vi "Sort Fcurve.vi"(0 "reference in":refnum<class "Force Curve_tdms.lvclass">, 5 "error in (no error)":errorcluster) -> (14 "reference out":refnum<class "Force Curve_tdms.lvclass">, 19 "error out":errorcluster)   [LabVIEW 2019, in "Force Curve_tdms.lvclass"]
uses:
  Force Curve_tdms.lvclass
  Signal In.ctl
  TDMS_DataHandler_class/property name combo box.ctl
  TDMS_DataHandler_class/TDMS_DataHandler.lvclass
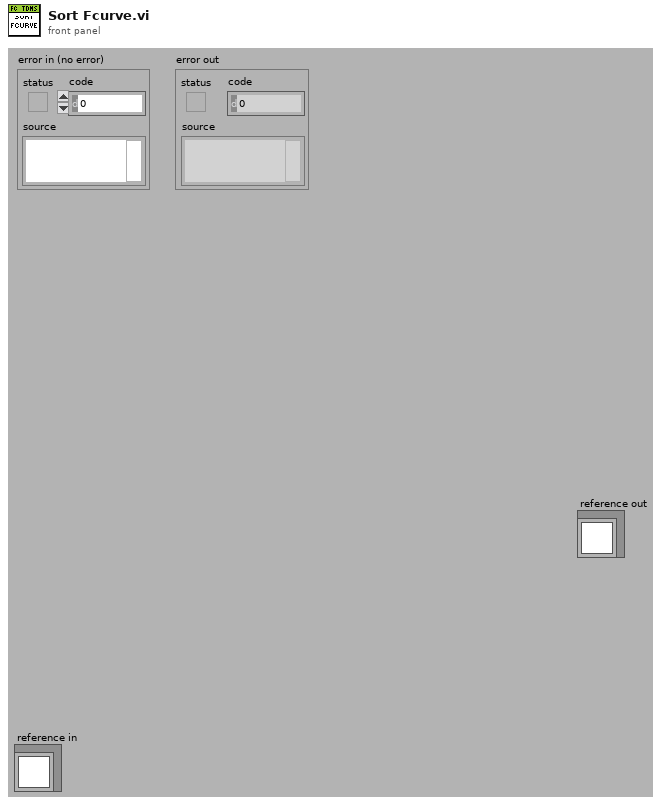
[diagram p1: front panel]
types:
  T1 = typedef "Force Curve_tdms.lvclass/Signal In.ctl" = enum16{"Deflection", "SensorIn", "MockOut", "ZstageOut"}
  T2 = typedef "TDMS_DataHandler.lvclass/property name combo box.ctl" = string
  T3 = typedef "Force Curve_tdms.lvclass/Fcurve Meta data analysis.ctl" = cluster{"dt (us)":dbl, "Dec Factor":dbl, "Z piezo Sensitivity (nm/V)":dbl, "K (N/m)":dbl, "Sp (V)":dbl, "Contact (ms)":dbl, "Zpos contact":dbl, "Vel_app (nm/s)":dbl, "Vel_ret (nm/s)":dbl, "deltaV (nm)":dbl, "Def_V0 (v)":dbl, "Decimating Factor":dbl}
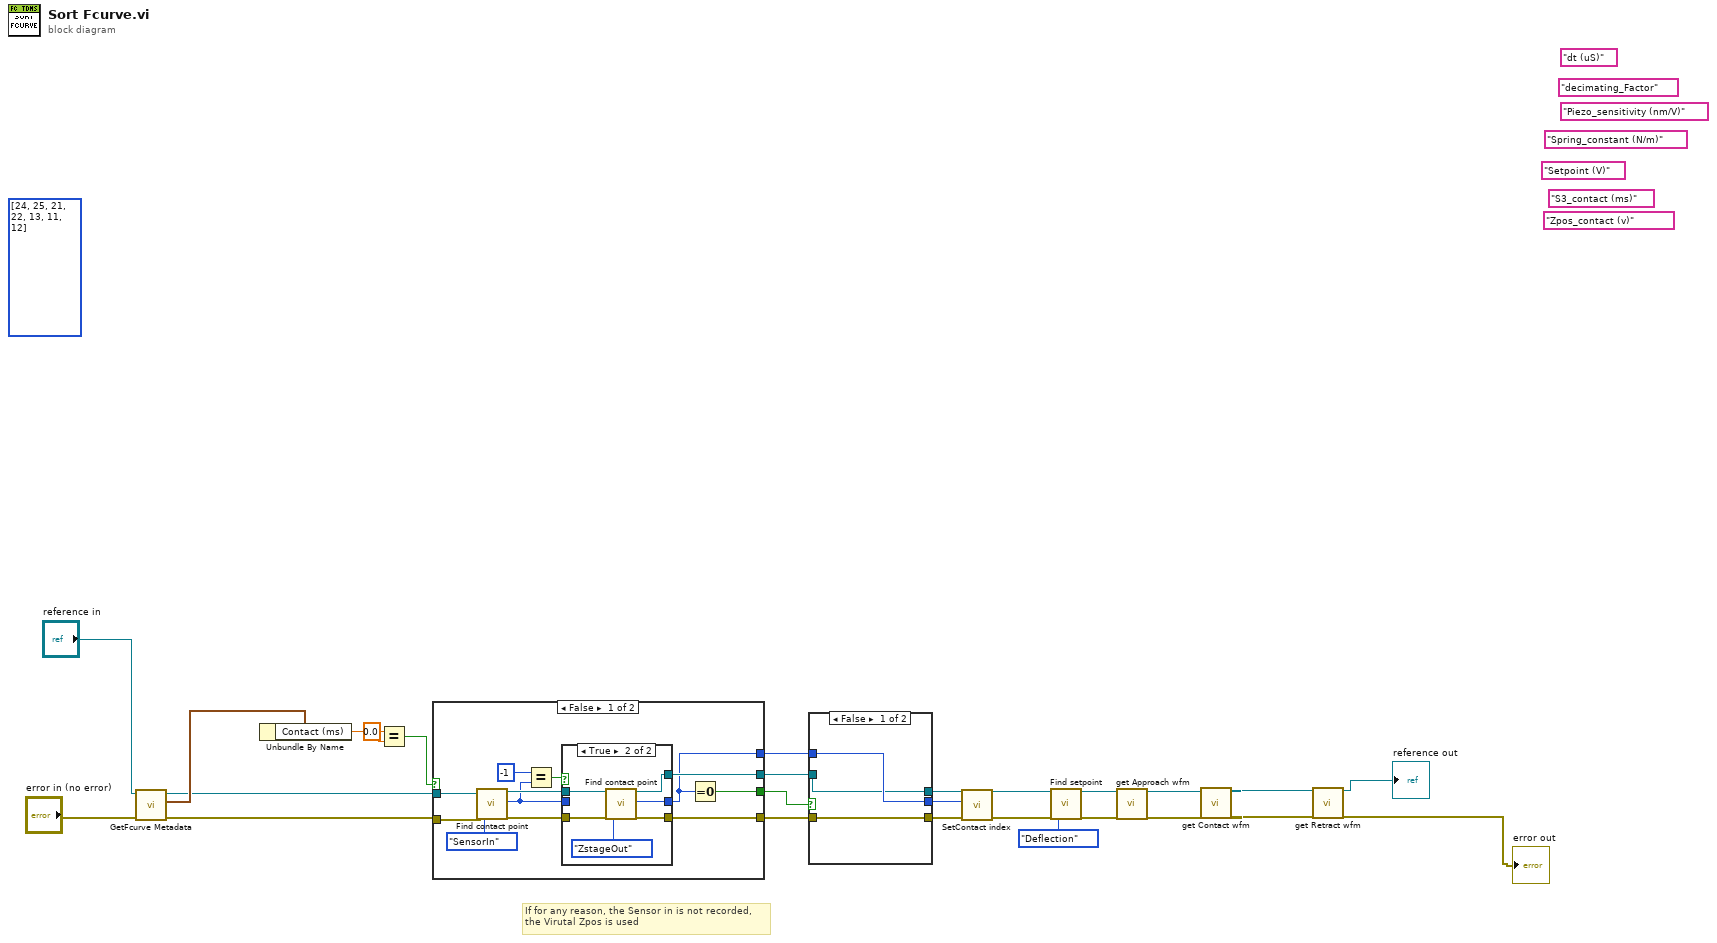
[diagram p0: block diagram]
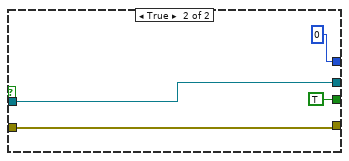
[diagram p3: hidden frame]
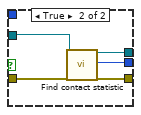
[diagram p4: hidden frame]
diagram:
  (unwired) i32[] [24, 25, 21, 22, 13, 11, 12] ("Array")
  (unwired) T2 "Setpoint (V)" ("Combo Box")
  (unwired) T2 "S3_contact (ms)" ("Combo Box")
  (unwired) T2 "Zpos_contact (v)" ("Combo Box")
  (unwired) T2 "Spring_constant (N/m)" ("Combo Box")
  (unwired) T2 "Piezo_sensitivity (nm/V)" ("Combo Box")
  (unwired) T2 "decimating_Factor" ("Combo Box")
  (unwired) T2 "dt (uS)" ("Combo Box")
  # "If for any reason, the Sensor in is not recorded,\nthe Virutal Zpos is used"
  n1 = call-dynamic "GetFcurve Metadata.vi"("error in (no error)"="error in (no error)", "reference in"="reference in") -> ("error out"=w18:errorcluster, "Fcurve Metadata"=w22:T3, "reference out"=w17:refnum<class "Force Curve_tdms.lvclass">)  [unwired: 7 in]
  n2 = Unbundle By Name(w22) -> ("Contact (ms)"=w21:dbl)
  n3 = Equal?(x=0.0, y=w21) -> (x = y?=w19:bool)
  n4 = case shown="False" w19 {
    tunnel: [w38 w51] -> w24
    tunnel: w18 -> [w37 w51]
    tunnel: [w36 TRUE] -> w23
    tunnel: [w28 0 ("Zpos index")] -> w11
    tunnel: w17 -> [w32 w48]
    tunnel: [w30 w48] -> w16
    frame False {
      n5 = call "Find contact point.vi"("reference in"=w32, "error in (no error)"=w37, "Signal in"=Signal_In."SensorIn") -> ("reference out"=w31:refnum<class "Force Curve_tdms.lvclass">, "contact index"=w27:i32, "error out"=w33:errorcluster)  [unwired: 14 in]
      n6 = Equal?(x=-1, y=w27) -> (x = y?=w34:bool)
      n7 = case shown="True" w34 {
        tunnel: w33 -> [w41 w47]
        tunnel: [w41 w46] -> w38
        tunnel: [w40 w45] -> w28
        tunnel: w27 -> [w40 _]
        tunnel: w31 -> [w39 w44]
        tunnel: [w39 w43] -> w30
        frame False {
        }
        frame True {
          n8 = call "Find contact point.vi"("reference in"=w44, "error in (no error)"=w47, "Signal in"=Signal_In."ZstageOut") -> ("reference out"=w43:refnum<class "Force Curve_tdms.lvclass">, "contact index"=w45:i32, "error out"=w46:errorcluster)  [unwired: 14 in]
        }
      }
      n9 = Equal To 0?(x=w28) -> (x = 0?=w36:bool)
    }
    frame True {
    }
  }
  n10 = case shown="False" w23 {
    tunnel: w24 -> [w53 w59]
    tunnel: [w53 w58] -> w5
    tunnel: [w54 w57] -> w2
    tunnel: w11 -> [w54 _]
    tunnel: w16 -> [w52 w56]
    tunnel: [w52 w55] -> w7
    frame False {
    }
    frame True {
      n11 = call "Find contact statistic.vi"("reference in"=w56, "error in (no error)"=w59) -> ("reference out"=w55:refnum<class "Force Curve_tdms.lvclass">, "contact point index out"=w57:i32, "error out"=w58:errorcluster)  [unwired: 15 in]
    }
  }
  n12 = call-dynamic "SetContact index.vi"("error in (no error)"=w5, "Contact index"=w2, "reference in"=w7) -> ("error out"=w4:errorcluster, "reference out"=w6:refnum<class "Force Curve_tdms.lvclass">)  [unwired: 7 in]
  n13 = call "Find setpoint.vi"("reference in"=w6, "error in (no error)"=w4, "Signal in"=Signal_In."Deflection") -> ("reference out"=w1:refnum<class "Force Curve_tdms.lvclass">, "error out"=w3:errorcluster)  [unwired: 14 in, 1 out]
  n14 = call-dynamic "get Approach wfm.vi"("reference in"=w1, "error in (no error)"=w3) -> ("reference out"=w15:refnum<class "Force Curve_tdms.lvclass">, "error out"=w14:errorcluster)  [unwired: 15 in, 1 out]
  n15 = call-dynamic "get Contact wfm.vi"("reference in"=w15, "error in (no error)"=w14) -> ("reference out"=w13:refnum<class "Force Curve_tdms.lvclass">, "error out"=w12:errorcluster)  [unwired: 15 in, 1 out]
  n16 = call-dynamic "get Retract wfm.vi"("reference in"=w13, "error in (no error)"=w12) -> ("reference out"=→"reference out":refnum<class "Force Curve_tdms.lvclass">, "error out"=→"error out":errorcluster)  [unwired: 15 in, 1 out]
